vi "find guid and channel pair.vi"(9 "channel name":string, 10 "Module GUID":string, 11 "listing":T1) -> (3 "index":i32)   [LabVIEW 2013, in "engine configuration.lvclass"]
uses:
  engine configuration.lvclass
  module channel pairings.ctl
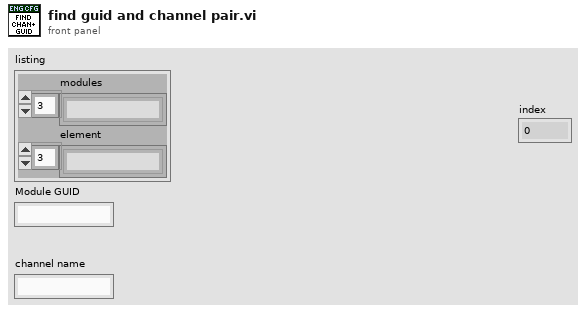
[diagram p1: front panel]
types:
  T1 = typedef "engine configuration.lvclass/module channel pairings.ctl" = cluster{"modules":string[], "element":string[]}
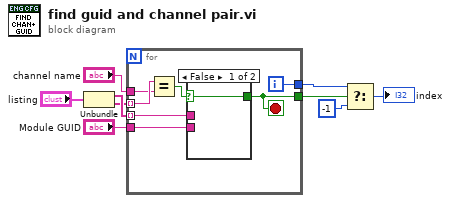
[diagram p0: block diagram]
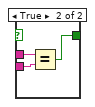
[diagram p2: hidden frame]
diagram:
  n1 = Unbundle("listing") -> ("modules"=w8:string[], "element"=w7:string[])
  n2 = for {
    tunnel: w8 -> [w13] mode=indexing
    tunnel: w7 -> [w16] mode=indexing
    tunnel: "channel name" -> [w15]
    tunnel: "Module GUID" -> [w12]
    tunnel: [w11] -> w4
    tunnel: [w10] -> w3
    i -> [w10]
    stop <- w11 stop-if-true
    n3 = Equal?(x=w16, y=w15) -> (x = y?=w14:bool)
    n4 = case shown="False" w14 {
      selector: w14 -> [w17 _]
      tunnel: w13 -> [_ w20]
      tunnel: w12 -> [_ w19]
      tunnel: [w17 w18] -> w11
      frame False {
      }
      frame True {
        n5 = Equal?(x=w20, y=w19) -> (x = y?=w18:bool)
      }
    }
  }
  n6 = Select(t=w3, s=w4, f=-1) -> (s? t:f=→"index":i32)
